vi "Extract_Patches_2d.vi"(8 "error in":errorcluster caption="entrée d'erreur", 10 "Image":string[][](array[string]), 11 "extract_patches_2d":T2={"patch_size"={"patch_height"=0, "patch_width"=0}, "max_patches"="None", "random_state"=-1} {"random_state" min=-1}) -> (0 "error out":errorcluster caption="sortie d'erreur", 3 "Data":T1)   [LabVIEW 2020]
doc: "Reshape a 2D image into a collection of patches\n\nThe resulting patches are allocated in a dedicated array.\n\nParameters :\n\n- image : ndarray of shape (image_height, image_width) or (image_height, image_width, n_channels)\nThe original image data. For color images, the last dimension specifies the channel: a RGB image would have n_channels=3.\n\n- patch_size : tuple of int (patch_height, patch_width)\nThe dimensions of one patch.\n\n- max_patches : int or float, default=None\nThe maximum number of patches to extract. If max_patches is a float between 0 and 1, it is taken to be a proportion of the total number of patches.\n\n- random_state : int, RandomState instance, default=None=-1\nDetermines the random number generator used for random sampling when max_patches is not None. Use an int to make the randomness deterministic. See Glossary.\n\nReturns : \n\n- patches : array of shape (n_patches, patch_height, patch_width) or (n_patches, patch_height, patch_width, n_channels)\nThe collection of patches extracted from the image, where n_patches is either max_patches or the total number of patches that can be extracted."
uses:
  Extract_Patches_2d.lvclass
panel:
  out "Extract_Patches_2d.lvclass":refnum<class "Extract_Patches_2d.lvclass">
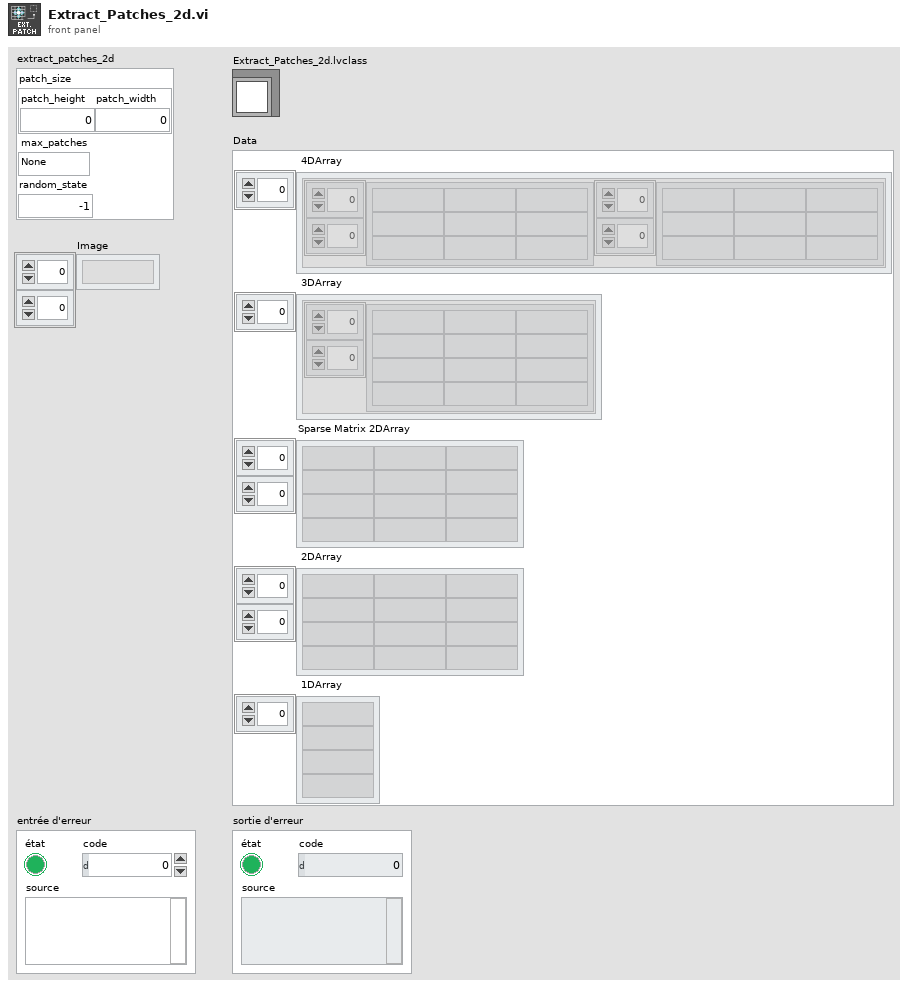
[diagram p1: front panel]
types:
  T1 = cluster{" 4DArray":cluster{"1":string[][], "2":string[][]}[], " 3DArray":cluster{"Tableau":string[][]}[], "Sparse Matrix 2DArray":string[][], " 2DArray":string[][], " 1DArray":string[]}
  T2 = cluster{"patch_size":cluster{"patch_height":i32, "patch_width":i32}, "max_patches":string, "random_state":i32}
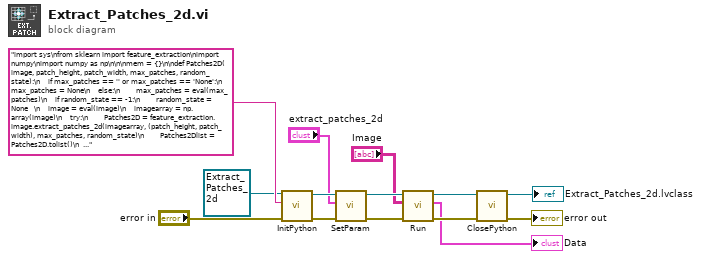
[diagram p0: block diagram]
diagram:
  n1 = call-dynamic "InitPython.vi"("error in (no error)"="error in", "Python Instruction"="import sys\nfrom sklearn import feature_extraction\nimport numpy\nimport numpy as np\n\n\nmem = {}\n\ndef Patches2D( image, patch_height, patch_width, max_patches, random_state):\n    if max_patches == '' or max_patches == 'None':\n        max_patches = None\n    else:\n        max_patches = eval(max_patches)\n    if random_state == -1:\n        random_state = None   \n    image = eval(image)\n    imagearray = np.array(image)\n    try:\n        Patches2D = feature_extraction.image.extract_patches_2d(imagearray, (patch_height, patch_width), max_patches, random_state)\n        Patches2Dlist = Patches2D.tolist()\n        return str(Patches2Dlist)\n    except:\n        erreur = sys.exc_info()\n        typerr = u\"%s\" % (erreur[0])\n        typerr = typerr[typerr.find(\"'\")+1:typerr.rfind(\"'\")]\n        msgerr = u\"%s\" % (erreur[1])\n        message = str('/!\\\\ {0} : {1}'. format(typerr,msgerr))\n        return message", "Scikit-learn en entrée"=refnum<class "Extract_Patches_2d.lvclass"> refnum ("Extract_Patches_2d.lvclass")) -> ("error out"=w11:errorcluster, "Scikit-learn en sortie"=w10:refnum<class "Extract_Patches_2d.lvclass">)  [unwired: 7 in]
  n2 = call-dynamic "SetParam.vi"("error in (no error)"=w11, "extract_patches_2d"="extract_patches_2d", "Extract_Patches_2d.lvclass"=w10) -> ("error out"=w5:errorcluster, "Extract_Patches_2d.lvclass"=w6:refnum<class "Extract_Patches_2d.lvclass">)  [unwired: 7 in]
  n3 = call-dynamic "Run.vi"("error in (no error)"=w5, "Image"="Image", "Extract_Patches_2d.lvclass"=w6) -> ("error out"=w2:errorcluster, "Data"=→"Data":T1, "Extract_Patches_2d.lvclass"=w3:refnum<class "Extract_Patches_2d.lvclass">)  [unwired: 6 in]
  n4 = call-dynamic "ClosePython.vi"("error in (no error)"=w2, "Scikit-learn en entrée"=w3) -> ("error out"=→"error out":errorcluster, "Scikit-learn en sortie"=→"Extract_Patches_2d.lvclass":refnum<class "Extract_Patches_2d.lvclass">)  [unwired: 8 in]
